vi "Open Default App Reference.vi"(8 "error in (no error)":errorcluster) -> (0 "error out":errorcluster, 2 "VI Server Configured?":bool, 3 "App Ref":refnum<vi>)   [LabVIEW 2020, in "MacroAssert.lvlib"]
doc: "Opens and outputs a reference to the default application instance, which can take on several possible values depending on the way in which the tool was launched."
uses:
  MacroAssert.lvlib
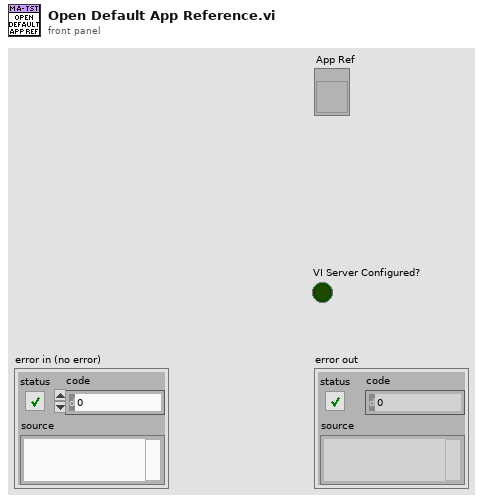
[diagram p1: front panel]
types:
  T1 = enum32{"invalid app kind", "Development System", "Run Time System", "Student Edition", "Embedded LabVIEW", "Evaluation", "Custom"}
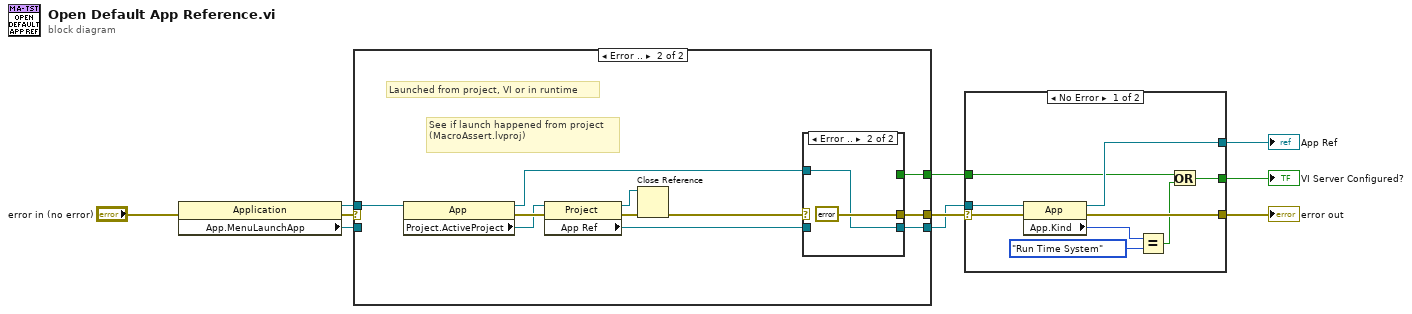
[diagram p0: block diagram]
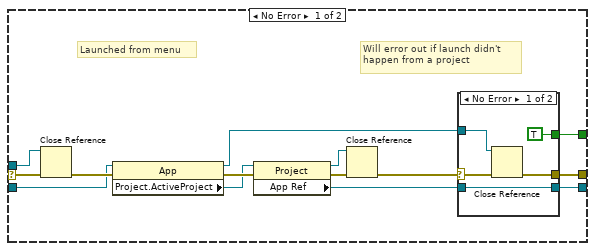
[diagram p2: hidden frame]
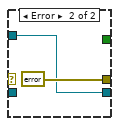
[diagram p3: hidden frame]
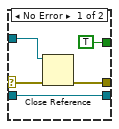
[diagram p4: hidden frame]
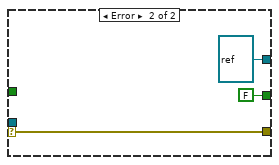
[diagram p5: hidden frame]
diagram:
  n1 = property class="Application"(error in="error in (no error)") -> (reference out=w4:refnum<vi>, error out=w9:errorcluster, "App.MenuLaunchApp"=w5:refnum<vi>)  [unwired: 1 in]
  n2 = case shown="Error .." w9 {
    selector: w9 -> [w24 _]
    tunnel: [w13 w34] -> w3
    tunnel: w5 -> [w16 _]
    tunnel: w4 -> [w18 w38]
    tunnel: [w19 w37] -> w7
    tunnel: [w11 w32] -> w1
    frame No Error {
      # "Will error out if launch didn't happen from a project"
      # "Launched from menu"
      n3 = Close Reference(reference=w18, error in (no error)=w24) -> (error out=w23:errorcluster)
      n4 = property class="App"(reference=w16, error in=w23) -> (reference out=w15:refnum<vi>, error out=w22:errorcluster, "Project.ActiveProject"=w17:refnum<vi>)
      n5 = property class="Project"(reference=w17, error in=w22) -> (reference out=w14:refnum<vi>, error out=w21:errorcluster, "App Ref"=w12:refnum<vi>)
      n6 = Close Reference(reference=w14, error in (no error)=w21) -> (error out=w20:errorcluster)
      n7 = case shown="No Error" w20 {
        selector: w20 -> [w29 _]
        tunnel: w15 -> [w27 w30]
        tunnel: [w28 errorcluster {"status"=FALSE, "code"=0, "source"=""} ("error out")] -> w19
        tunnel: [w26 w30] -> w13
        tunnel: w12 -> [w26 _]
        tunnel: [TRUE _] -> w11
        frame No Error {
          n8 = Close Reference(reference=w27, error in (no error)=w29) -> (error out=w28:errorcluster)
        }
        frame Error {
        }
      }
    }
    frame Error {
      # "Launched from project, VI or in runtime"
      # "See if launch happened from project (MacroAssert.lvproj)"
      n9 = property class="App"(reference=w38) -> (reference out=w33:refnum<vi>, error out=w42:errorcluster, "Project.ActiveProject"=w40:refnum<vi>)  [unwired: 1 in]
      n10 = property class="Project"(reference=w40, error in=w42) -> (reference out=w39:refnum<vi>, error out=w41:errorcluster, "App Ref"=w35:refnum<vi>)
      n11 = Close Reference(reference=w39, error in (no error)=w41) -> (error out=w36:errorcluster)
      n12 = case shown="Error .." w36 {
        selector: w36 -> [w47 _]
        tunnel: w33 -> [w45 w48]
        tunnel: [w46 errorcluster {"status"=FALSE, "code"=0, "source"=""} ("error out")] -> w37
        tunnel: [w44 w48] -> w34
        tunnel: w35 -> [w44 _]
        tunnel: [TRUE _] -> w32
        frame No Error {
          n13 = Close Reference(reference=w45, error in (no error)=w47) -> (error out=w46:errorcluster)
        }
        frame Error {
        }
      }
    }
  }
  n14 = case shown="No Error" w7 {
    selector: w7 -> [w58 w61]
    tunnel: w3 -> [w56 _]
    tunnel: [w57 w61] -> w10
    tunnel: [w55 refnum<vi> refnum ("application reference")] -> w6
    tunnel: [w52 FALSE] -> w2
    tunnel: w1 -> [w50 _]
    frame No Error {
      n15 = property class="App"(reference=w56, error in=w58) -> (reference out=w55:refnum<vi>, error out=w57:errorcluster, "App.Kind"=w54:T1)
      n16 = Equal?(x=w54, y=T1."Run Time System") -> (x = y?=w51:bool)
      n17 = Or(x=w50, y=w51) -> (x .or. y?=w52:bool)
    }
    frame Error {
    }
  }
  "error out" <- w10
  "App Ref" <- w6
  "VI Server Configured?" <- w2
